vi "Send_Notifier.vi"(9 "Stream Type":T1, 11 "navX Action":T2) -> ()   [LabVIEW 2015]
uses:
  _TypeDefs/Z900_navX_ActionTypeDef.ctl
  _TypeDefs/Z900_navX_SerialStreamTypeDef.ctl
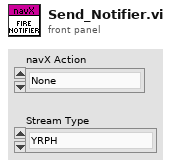
[diagram p1: front panel]
types:
  T1 = typedef "Z900_navX_SerialStreamTypeDef.ctl" = enum16{"YRPH", "Quaterinons", "Gyro/Raw", "AHRS", "AHRSAndPositioning"}
  T2 = typedef "Z900_navX_ActionTypeDef.ctl" = enum16{"None", "Halt", "Normal Read", "Update Serial Protocol", "Update Rate Htz", "Zero-Yaw", "Zero-Displacement", "Zero-Velocity"}
  T3 = typedef "Z900_navX_NotifyPacketTypeDef.ctl" = cluster{"navX Action":T2, "Data":variant, "Stream Type":T1}
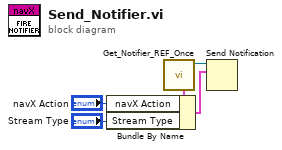
[diagram p0: block diagram]
diagram:
  n1 = call "Get_Notifier_REF_Once.vi"() -> ("notifier ref out"=w5:refnum<notifier>, "notification"=w4:T3)  [unwired: 10 in]
  n2 = Bundle By Name(cluster=w4, "navX Action"="navX Action", "Stream Type"="Stream Type") -> (w3:T3)
  n3 = Send Notification(notification=w3, notifier=w5) -> ()  [unwired: 1 in, 2 out]
